vi "Drive Fw for x feet.vi"(11 "Feet":dbl) -> (10 "Y-Axis":dbl)   [LabVIEW 2017]
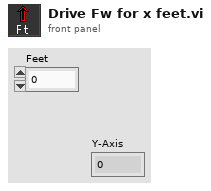
[diagram p1: front panel]
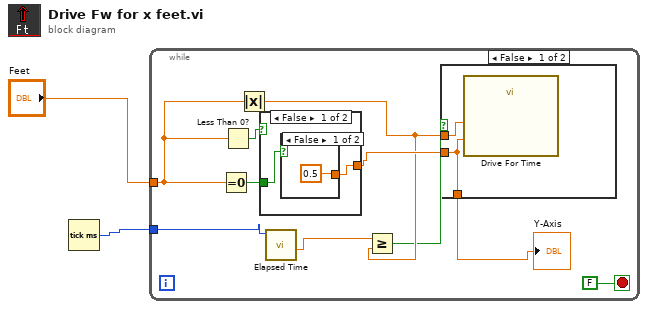
[diagram p0: block diagram]
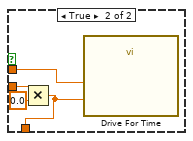
[diagram p2: hidden frame]
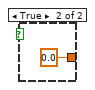
[diagram p3: hidden frame]
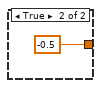
[diagram p4: hidden frame]
diagram:
  n1 = Tick Count (ms)() -> (millisecond timer value=w1:u32)
  n2 = while {
    tunnel: w1 -> [w9]
    tunnel: "Feet" -> [w4]
    stop <- FALSE stop-if-true
    n3 = Equal To 0?(x=w4) -> (x = 0?=w10:bool)
    n4 = Less Than 0?(x=w4) -> (x < 0?=w12:bool)
    n5 = Absolute Value(x=w4) -> (abs(x)=w7:dbl)
    n6 = case shown="False" w12 {
      tunnel: [w19 -0.5] -> w11
      tunnel: w10 -> [w20 _]
      frame False {
        n7 = case shown="False" w20 {
          tunnel: [0.5 0.0] -> w19
          frame False {
          }
          frame True {
          }
        }
      }
      frame True {
      }
    }
    n8 = call "Elapsed Time.vi"("Start Time"=w9) -> ("Elapsed Time"=w8:dbl)  [unwired: 10 in]
    n9 = Greater Or Equal?(x=w8, y=w7) -> (x >= y?=w6:bool)
    n10 = case shown="False" w6 {
      tunnel: w11 -> [w13 w17]
      tunnel: w7 -> [w14 w18]
      tunnel: [w13 w15] -> w3
      frame False {
        n11 = call "Drive For Time.vi"("Y"=w13, "Time(s)"=w14) -> ()  [unwired: 10 in]
      }
      frame True {
        n12 = Multiply(x=w17, y=0.0) -> (x*y=w15:dbl)
        n13 = call "Drive For Time.vi"("Y"=w15, "Time(s)"=w18) -> ()  [unwired: 10 in]
      }
    }
    "Y-Axis" <- w3
  }
